vi "commander6.vi"() -> ()   [LabVIEW 2015]
uses:
  G_DATA.vi
  G_LCM.vi
  G_VEH.vi
  G_NAV.vi
  G_PATH.vi
  G_SEN.vi
  <vilib>/addons/control/pid/pid.llb/PID (DBL).vi
  <vilib>/addons/control/pid/NI_PID_pid.lvlib
panel:
  in  "handle":dbl
  in  "shifthold":dbl=0.0025
  out "String":string="콜 서비스 대기 중"
  out "EURECAR_VISION":T1
  out "count":i32
  out "P2V Sign":picture[](array[picture])=[bytes[7530], bytes[7530], bytes[7530], bytes[7530]]
  out "Array 2":picture[](array[picture])
  out "sign 2":picture[](array[picture])
  out "sign":picture[](array[picture])
  in  "TTL":bool
  in  "Steering gain":dbl=0.8
  out "obs shift":dbl format="%.2f"
  in  "lane keep":bool
  in  "replay":bool
  in  "x":dbl min=-5.0 max=5.0 step=1.0
  out "lane_shift":dbl=0.06529975046455076
  out "display":u32=10
  out "control":u32=10
  out "update":bool=TRUE
  in  "save lcm":bool
  out "LCM Recv Data":string="GGA_2\t266\rSDT_GPS_DATA\t268\rGGA_1\t268\rRMC_2\t259\rRMC_1\t262\rEYE_RAW_T\t537\rPATH_T\t1344\rIBEO_2202_T\t672\rPOS_T\t3572\rCON_T\t4009\rCAN_T\t4707\r"
  out "GPS DATA 2":T2={"type"="WAAS", "x_lcc"=-395.2637182511565, "y_lcc"=-852.8277788987846, "latdev"=0.99, "londev"=0.99, "sats"=11, "gps_l1_ranges"=0, "gps_l1_mask_ranges"=0, "gps_l2_mask_ranges"=0, "Heading"=151.74409645131422, "lon"=127.35651, "lat"=36.36776, "time"="15:03:34.8", "hgps"=151.54, "lag"=0.0, "MAP"="KAIST"} {"lag" format="%#_5g"; "hgps" format="%#_5g"; "lat" format="%#_11g"; "lon" format="%#_11g"; "Heading" format="%#_5g"; "latdev" format="%#_4g"; "londev" format="%#_4g"}
  in  "Obs":bool=TRUE
  in  "Log":bool
  out "path":u32=10
  out "sensor":u32=10 format="%02.0f"
  out "Speed limit":dbl=20.0
  out "collision":bool
  in  "Load Path":bool
  in  "Max. Vel.":dbl=20.0 min=-5.0 max=120.0 step=5.0
  in  "RESET PATH":bool
  out "col":i16(graph)
  out "stop":bool
  in  "Reverse":bool
  in  "STOP":bool
  out "Waveform Chart 4":cluster{"auto":i16, "run":i16}(graph)={"auto"=1, "run"=0}
  out "Waveform Chart 3":cluster{"Steer_input":dbl, dbl, "handle":dbl}(graph)
  out "Waveform Chart 2":T3(graph)={"VS_des"=0.0, "VS_can"=31.498562500000002, "VS_des"=20.0}
  out "Heading":cluster{"Heading":dbl, "hgps":dbl}(graph)={"Heading"=151.74409645131422, "hgps"=151.54}
  out "XY Graph 2":cluster{"Y":dbl[], "Y":dbl[]}[](graph)=[{"Y"=[-395.3040396828474], "Y"=[-852.7527551292769]}, {"Y"=array[29298 elements], "Y"=array[29298 elements]}, {"Y"=array[29298 elements], "Y"=array[29298 elements]}, {"Y"=[-390.58210518912017], "Y"=[-861.284610912867]}]
  out "Gauge":cluster{dbl, dbl, dbl}(knob)={0.0, 31.498562500000002, 20.0} scale=-20.0..140.0
  out "Meter":cluster{dbl, dbl, dbl}(knob)={-3.5333877271700453, -5.2, -7.217874503679048} scale=-550.0..550.0
  out "XY Graph":cluster{"Y":dbl[], "Y":dbl[]}[](graph)=[{"Y"=array[11233 elements], "Y"=array[11233 elements]}, {"Y"=[-0.0, 0.0027755521495791413, 0.011103235155417224, 0.024986130588096955, 0.04442938073793812, 0.0694401981527264, 0.10002787904836907, 0.13620382065079895, 0.17798154254490584, 0.22537671212434418, 0.2784071742547809, 0.3370929852830926, 0.40145645154536425, 0.4715221725490224, 0.5473170890276435, 0.6288705360921867, 0.7162143017295008, 0.8093826909282242, 0.9084125957438758, 1.0133435716494645, 1.1242179205557647, 1.2410807809266515, 1.3639802254602955, 1.4929673668571652, 1.6280964722509026, 1.769425086939485, 1.9170141681219874, 2.0709282294217246, 2.2312354970611636, 2.3980080786478197, 2.5713221456362234], "Y"=[0.0, 0.5, 1.0, 1.5, 2.0, 2.5, 3.0, 3.5, 4.0, 4.5, 5.0, 5.5, 6.0, 6.5, 7.0, 7.5, 8.0, 8.5, 9.0, 9.5, 10.0, 10.5, 11.0, 11.5, 12.0, 12.5, 13.0, 13.5, 14.0, 14.5, 15.0]}, {"Y"=[-0.40885366553013214], "Y"=[0.1442103688222703]}, {"Y"=array[212 elements], "Y"=array[212 elements]}, {"Y"=[-0.925, -0.925, -0.925, -0.6775, -0.6775, -0.925, -0.925, -0.925, -0.925, -0.6775, -0.6775, -0.925, -0.925, -0.925, 0.9025, 0.9025, 0.9025, 0.6775, 0.6775, 0.9025, 0.9025, 0.9025, 0.9025, 0.6775, 0.6775, 0.9025, 0.9025, 0.9025, -0.925], "Y"=[-0.75, -0.224, 0.224, 0.224, -0.224, -0.224, 0.224, 2.415, 2.885, 2.885, 2.415, 2.415, 2.885, 3.5, 3.5, 2.885, 2.415, 2.415, 2.885, 2.885, 2.415, 0.224, -0.224, -0.224, 0.224, 0.224, -0.224, -0.75, -0.75]}, {"Y"=[0.0, 0.0, 0.0, 0.0, 0.0, 0.0, 0.0, 0.0, 0.0, 0.0], "Y"=[0.0, 0.5, 1.0, 1.5, 2.0, 2.5, 3.0, 3.5, 4.0, 4.5]}, {"Y"=[1.41796875, 1.3798326583616436, 1.3415997434556484, 1.3032752327956258, 1.2648643538951874, 1.226372334267944, 1.1878044014275073, 1.1491657828874886, 1.110461706161499, 1.07169739876315], "Y"=[0.0, 0.5, 1.0, 1.5, 2.0, 2.5, 3.0, 3.5, 4.0, 4.5]}, {"Y"=[-2.5234375, -2.5105986626297234, -2.4915998479127883, -2.466420726940036, -2.4350409708023073, -2.3974402505904435, -2.3535982373952864, -2.303494602307677, -2.247109016418457, -2.184421150818467], "Y"=[0.0, 0.5, 1.0, 1.5, 2.0, 2.5, 3.0, 3.5, 4.0, 4.5]}, {"Y"=[0.0, 0.0, 0.0, 0.0, 0.0, 0.0, 0.0, 0.0, 0.0, 0.0, 0.0, 0.0, 0.0, 0.0, 0.0, 0.0, 0.0, 0.0, 0.0, 0.0], "Y"=[0.0, 0.5, 1.0, 1.5, 2.0, 2.5, 3.0, 3.5, 4.0, 4.5, 5.0, 5.5, 6.0, 6.5, 7.0, 7.5, 8.0, 8.5, 9.0, 9.5]}]
  in  "Make WPT":bool
  # "e"
  # "V2I Traffic Signal"
  # "CNN\nSign\nDetection"
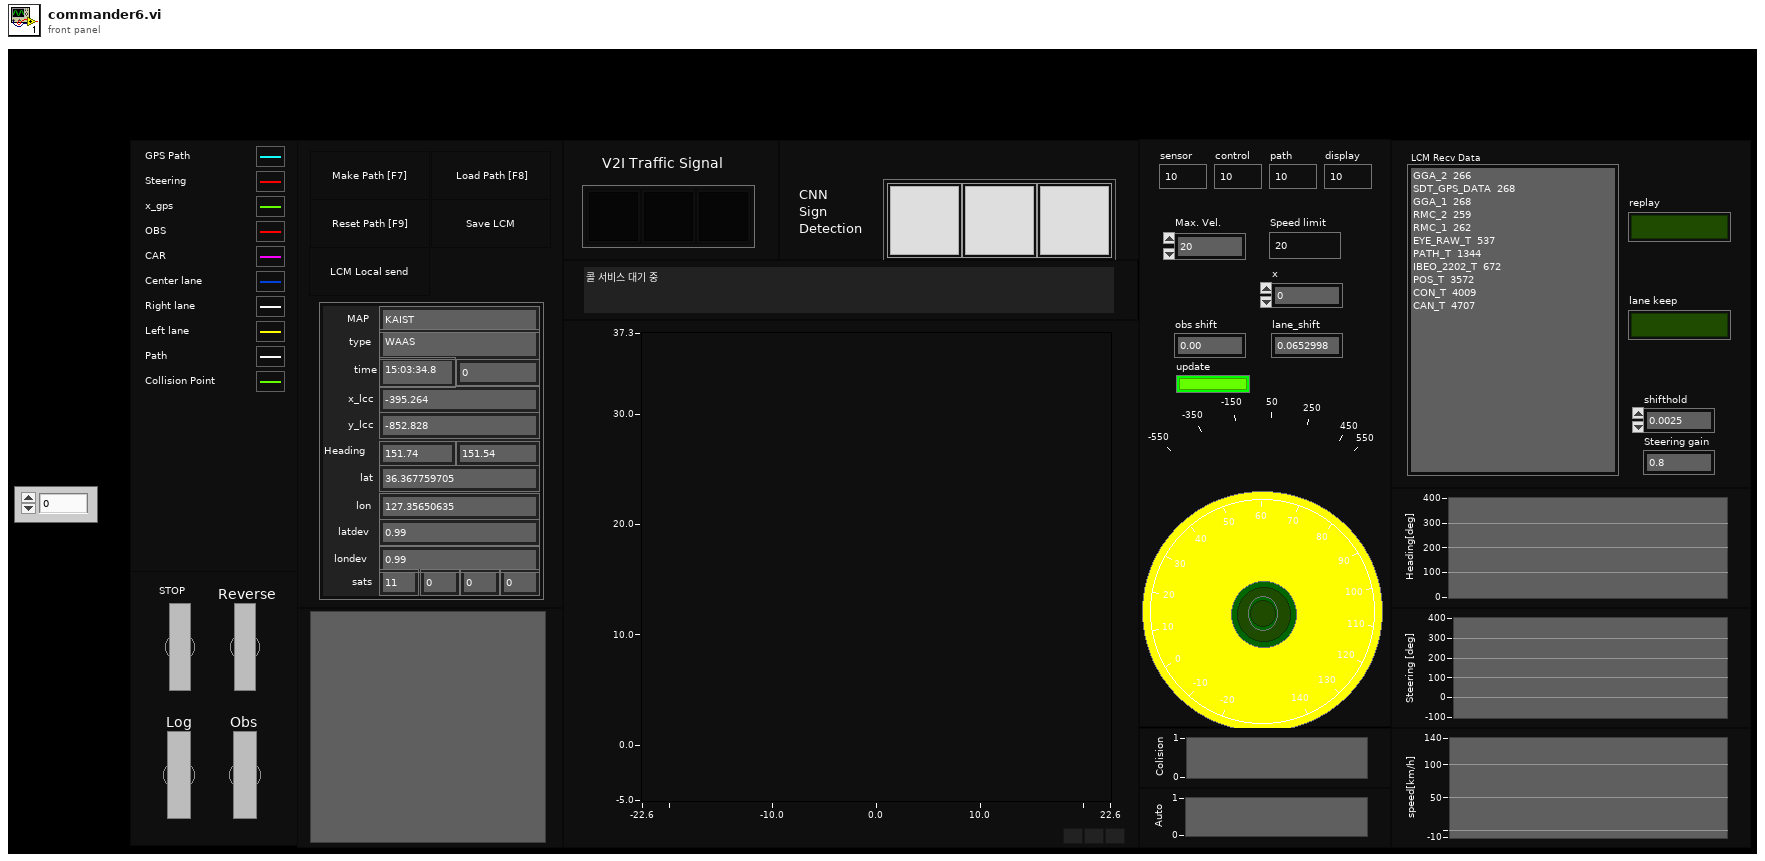
[diagram p1: front panel]
types:
  T1 = cluster{"hash":i64, "sys time":i64, "status":i32, "TS_num":i32, "TS_type":i32[], "TS_loc_x":dbl[], "TS_loc_y":dbl[]}
  T2 = cluster{"type":string, "x_lcc":dbl, "y_lcc":dbl, "latdev":sgl, "londev":sgl, "sats":u8, "gps_l1_ranges":u8, "gps_l1_mask_ranges":u8, "gps_l2_mask_ranges":u8, "Heading":dbl, "lon":sgl, "lat":sgl, "time":string, "hgps":dbl, "lag":dbl, "MAP":string}
  T3 = cluster{"VS_des":dbl, "VS_can":dbl, "VS_des":dbl}
  T4 = enum8{"Enabled", "Disabled", "Disabled and Grayed Out"}
  T5 = cluster{"proportional gain (Kc)":dbl, "integral time (Ti, min)":dbl, "derivative time (Td, min)":dbl}
  T6 = cluster{"idx":i32, "x":dbl, "y":dbl, "h":dbl, "x_path":dbl}
  T7 = cluster{"idx":i32, "x":dbl, "y":dbl, "hp":dbl, "x_path":dbl}
  T8 = cluster{"Steer_input":dbl, "Steer_output":dbl, "VS_des":dbl, "VS_can":dbl, "heading":dbl, "auto":bool, "run":bool, "x":dbl, "y":dbl}
  T9 = cluster{"X":cluster{"idx":i32, "x":dbl, "y":dbl, "h":dbl, "x_path":dbl}}[]
  T10 = typedef "imagedata.ctl" = cluster{"image type":i32, "image depth":i32, "image":u8[], "mask":u8[], "colors":u32[], "Rectangle":cluster{"left":i16, "top":i16, "right":i16, "bottom":i16}}
  T11 = cluster{"hash":i64, "sys time":i64, "s_lat":dbl, "s_lon":dbl, "d_lat":dbl, "d_lon":dbl, "Message":i64}
  T12 = cluster{"GPSTime":dbl, "attitude[2]":dbl, "lcc[0]":dbl, "lcc[1]":dbl, "heading_GPS":dbl}
  T13 = cluster{"Minimum":dbl, "Minimum":dbl, "Minimum":dbl, "Minimum":dbl, "Minimum":dbl}
  T14 = cluster{"X":cluster{"c_idx":i32, "xc":dbl, "yc":dbl, "hc":dbl, "xc_path":dbl}}[]
  T15 = cluster{"hash":i64, "sys time":i64, "time":dbl, "x":dbl, "y":dbl, "h":dbl, "numSV":i32, "postype":i32, "lag":i32, "hordev":dbl, "lat":dbl, "lon":dbl, "hgt":dbl, "map_idx":i32}
  T16 = cluster{"identifier":u32, "timestamp":timestamp, "payload":u8[]}
  T17 = cluster{"hash":i64, "sys time":i64, "size":i32, "data":u8[]}
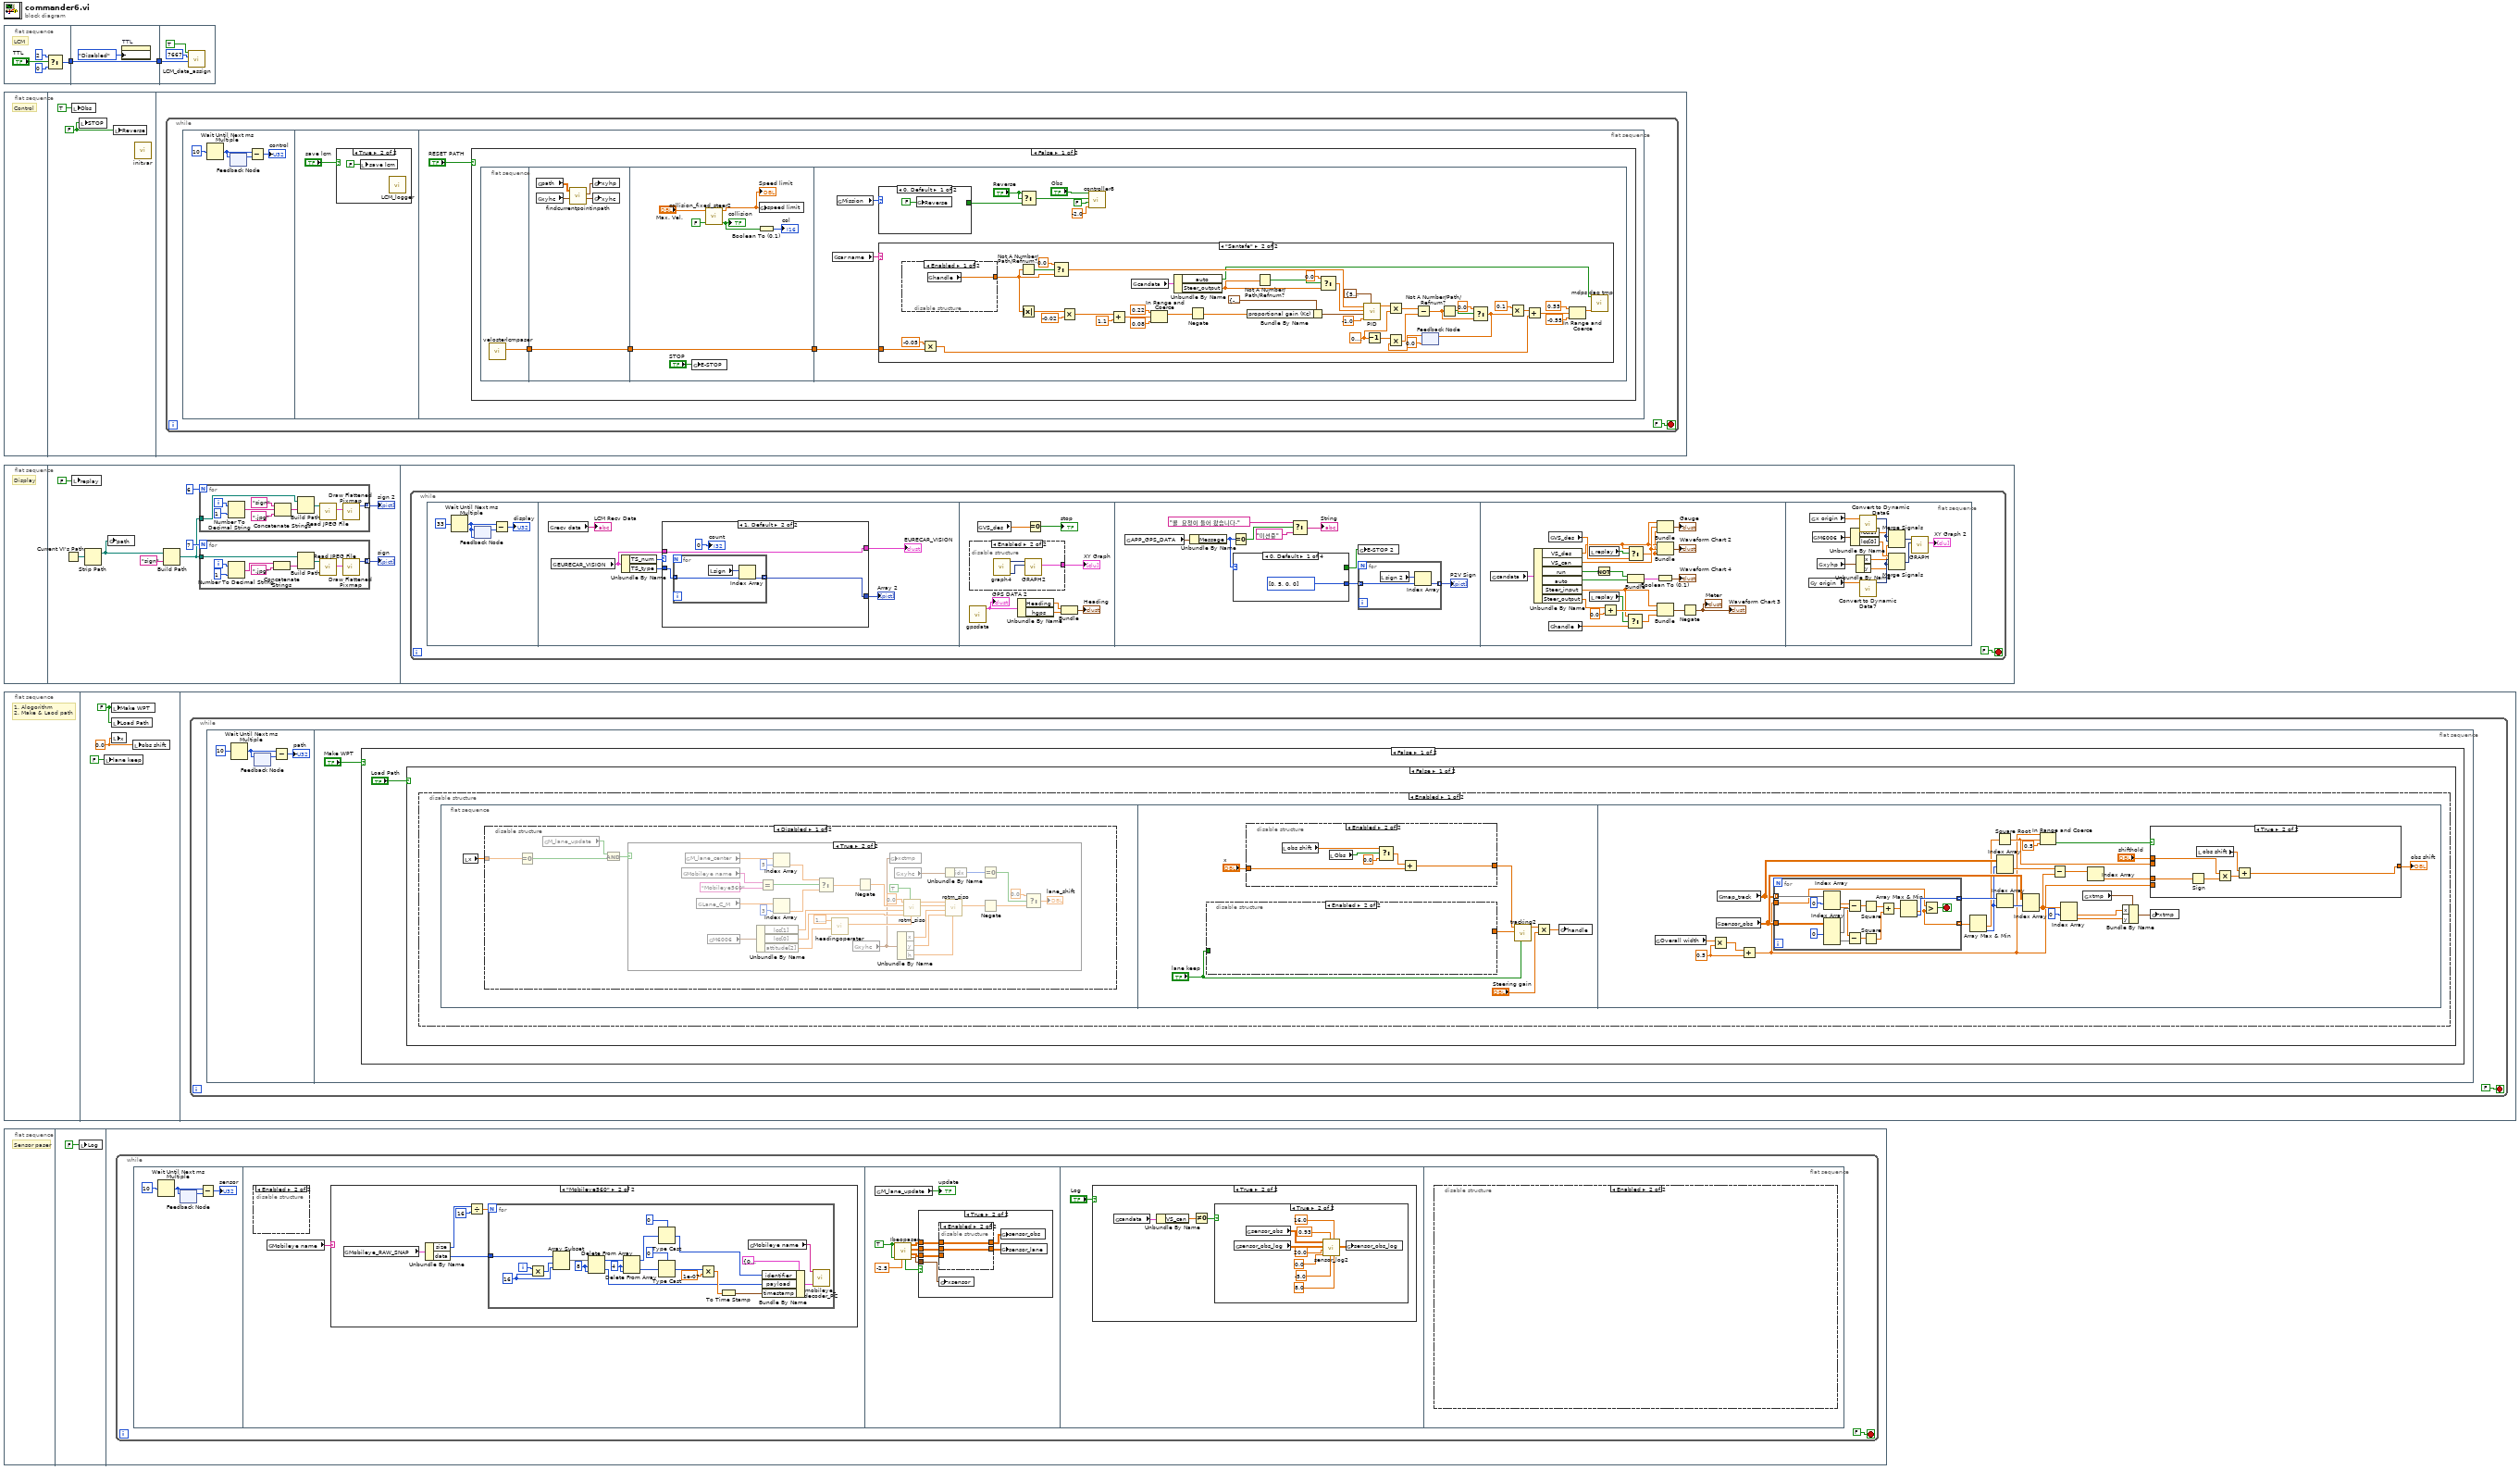
[diagram p0: block diagram]
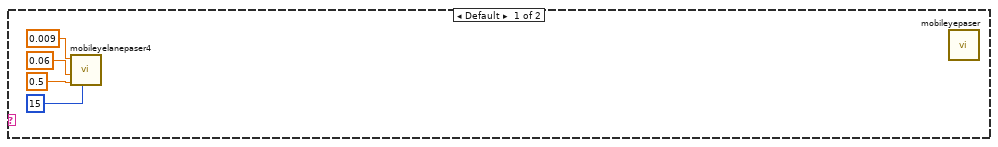
[diagram p2: hidden frame]
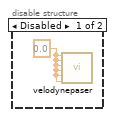
[diagram p3: hidden frame]
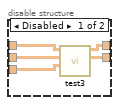
[diagram p5: hidden frame]
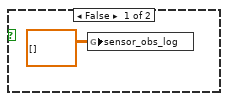
[diagram p6: hidden frame]
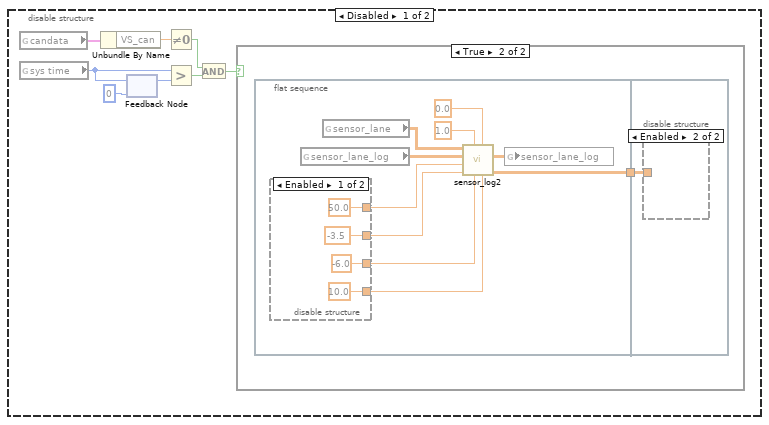
[diagram p8: hidden frame]
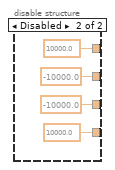
[diagram p10: hidden frame]
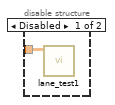
[diagram p11: hidden frame]
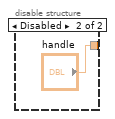
[diagram p14: hidden frame]
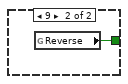
[diagram p15: hidden frame]
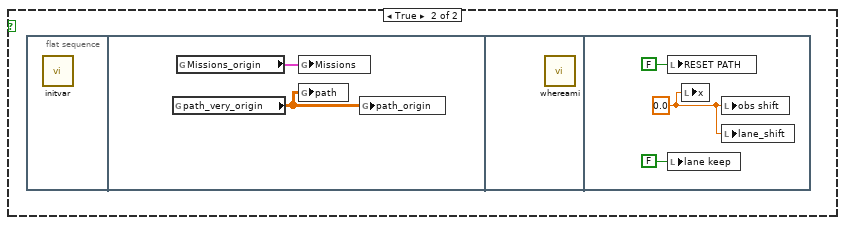
[diagram p16: hidden frame]
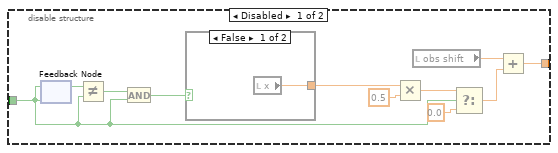
[diagram p19: hidden frame]
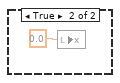
[diagram p20: hidden frame]
diagram:
  n1 = flat-sequence {
    tunnel: [w3] -> w1
    tunnel: [w8] -> w2
    tunnel: w1 -> [w8]
    tunnel: w2 -> [w11]
    frame #0 {
      # "LCM"
      n2 = Select(t=u16 2 ("time-to-live"), s="TTL", f=u16 0 ("time-to-live")) -> (s? t:f=w3:u16)
    }
    frame #1 {
      n3 = property on="TTL" class="Bool (strict)"("DisabledEnum"=T4."Disabled" ("Disabled")) -> ()  [unwired: 2 in, 2 out]
    }
    frame #2 {
      n4 = call "LCM_data_assign.vi"("time-to-live"=w11, "port"=u16 7667, "velodyne enable"=TRUE) -> ()  [unwired: 9 in]
    }
  }
  n5 = flat-sequence {
    frame #0 {
      # "Control"
    }
    frame #1 {
      w13 = FALSE ("LCM")
      n6 = local write "Obs"(TRUE ("obs")) -> ()
      n7 = local write "STOP"(w13) -> ()
      n8 = local write "Reverse"(w13) -> ()
      n9 = call "initvar.vi"() -> ()  [unwired: 12 in]
    }
    frame #2 {
      n10 = while {
        stop <- FALSE ("Loop 1") stop-if-true
        n11 = flat-sequence {
          frame #0 {
            n12 = Wait Until Next ms Multiple(millisecond multiple=u32 10 ("milliseconds to wait")) -> (millisecond timer value=w15:u32)
            n13 = feedback #1() -> (w16:u32)  [unwired: 1 in]
            n14 = feedback-in #1(w15) -> ()
            n15 = Subtract(x=w15, y=w16) -> (x-y=→"control":u32)
          }
          frame #1 {
            n16 = case shown="True" "save lcm" {
              frame False {
              }
              frame True {
                n17 = local write "save lcm"(FALSE ("save lcm")) -> ()
                n18 = call "LCM_logger.vi"() -> ()  [unwired: 12 in]
              }
            }
          }
          frame #2 {
            n19 = case shown="False" "RESET PATH" {
              frame False {
                n20 = flat-sequence {
                  tunnel: [w25] -> w24
                  tunnel: w24 -> [w26]
                  tunnel: [w26] -> w23
                  tunnel: w23 -> [w32]
                  tunnel: [w32] -> w22
                  tunnel: w22 -> [w40]
                  frame #0 {
                    n21 = call "velosterlcmpaser.vi"() -> ("mdps torque"=w25:dbl)  [unwired: 10 in, 1 out]
                  }
                  frame #1 {
                    n22 = global read "G_PATH.vi" "path"() -> (w28:dbl[][])
                    n23 = global read "G_VEH.vi" "xyhc"() -> (w29:T6)
                    n24 = call "findcurrentpointinpath.vi"("xyhc_in"=w29, "path_updated"=w28) -> ("xyhc_out"=w27:T6, "xyhp"=w30:T7)  [unwired: 8 in]
                    n25 = global write "G_VEH.vi" "xyhp"(w30) -> ()
                    n26 = global write "G_VEH.vi" "xyhc"(w27) -> ()
                  }
                  frame #2 {
                    n27 = global write "G_VEH.vi" "E-STOP"("STOP") -> ()
                    n28 = call "collision_fixed_steer2.vi"("obsclose"=FALSE, "Max. Vel."="Max. Vel.") -> ("collision"=w33:bool, "speed limit"=w31:dbl)  [unwired: 8 in]
                    "collision" <- w33
                    "Speed limit" <- w31
                    n29 = Boolean To (0,1)(Boolean=w33) -> (0, 1=→"col":i16)
                    n30 = global write "G_VEH.vi" "speed limit"(w31) -> ()
                  }
                  frame #3 {
                    n31 = global read "G_LCM.vi" "car name"() -> (w41:string)
                    n32 = global read "G_PATH.vi" "Mission"() -> (w46:i32)
                    n33 = case shown="0, Default" w46 {
                      tunnel: [_ w93] -> w43
                      frame 0, Default {
                        n34 = global write "G_VEH.vi" "Reverse"(FALSE ("Reverse")) -> ()
                      }
                      frame 9 {
                        n35 = global read "G_VEH.vi" "Reverse"() -> (w93:bool)
                      }
                    }
                    n36 = case shown="\"Santafe\"" w41 {
                      tunnel: w40 -> [_ w80]
                      frame "False", Default {
                      }
                      frame "Santafe" {
                        w69 = 0.6000000000000001 ("y")
                        n37 = disable-structure shown="Enabled" {
                          disable-tunnel: [w90 "handle"] -> w47
                          frame Enabled {
                            n38 = global read "G_VEH.vi" "handle"() -> (w90:dbl)
                          }
                          frame Disabled {
                          }
                        }
                        n39 = Multiply(x=-0.05 ("x 5"), y=w80) -> (x*y=w78:dbl)
                        n40 = Not A Number/Path/Refnum?(number/path/refnum=w47) -> (NaN/Path/Refnum?=w72:bool)
                        n41 = Absolute Value(x=w47) -> (abs(x)=w63:dbl)
                        n42 = Select(t=0.0, s=w72, f=w47) -> (s? t:f=w71:dbl)
                        n43 = Multiply(x=w63, y=-0.02) -> (x*y=w61:dbl)
                        n44 = Add(x=w61, y=1.1) -> (x+y=w59:dbl)
                        n45 = global read "G_VEH.vi" "candata"() -> (w89:T8)
                        n46 = In Range and Coerce(upper limit=0.22, x=w59, lower limit=0.08) -> (coerced(x)=w56:dbl)  [unwired: 1 out]
                        n47 = Unbundle By Name(w89) -> ("auto"=w48:bool, "Steer_output"=w75:dbl)
                        n48 = Negate(x=w56) -> (-x=w54:dbl)
                        n49 = Bundle By Name(cluster=T5 {"proportional gain (Kc)"=-0.1, "integral time (Ti, min)"=0.0, "derivative time (Td, min)"=0.0} ("PID gains"), "proportional gain (Kc)"=w54) -> (w53:T5)
                        n50 = Not A Number/Path/Refnum?(number/path/refnum=w75) -> (NaN/Path/Refnum?=w77:bool)
                        n51 = Select(t=0.0, s=w77, f=w75) -> (s? t:f=w74:dbl)
                        n52 = call-poly <vilib>:"PID.vi"("output range"=cluster{"output high":dbl, "output low":dbl} {"output high"=5.0, "output low"=-5.0}, "dt (s)"=-1.0, "PID gains"=w53, "process variable"=w74, "setpoint"=w71) -> ("output"=w70:dbl)  [unwired: 5 in, 1 out]
                        n53 = Decrement(x=w69) -> (x-1=w68:dbl)
                        n54 = Multiply(x=w70, y=w69) -> (x*y=w65:dbl)
                        n55 = feedback #2(0.0) -> (w67:dbl)
                        n56 = Multiply(x=w68, y=w67) -> (x*y=w66:dbl)
                        n57 = Subtract(x=w65, y=w66) -> (x-y=w50:dbl)
                        n58 = Not A Number/Path/Refnum?(number/path/refnum=w50) -> (NaN/Path/Refnum?=w52:bool)
                        n59 = Select(t=0.0, s=w52, f=w50) -> (s? t:f=w49:dbl)
                        n60 = feedback-in #2(w49) -> ()
                        n61 = Multiply(x=0.1 ("x 2"), y=w49) -> (x*y=w79:dbl)
                        n62 = Add(x=w79, y=w78) -> (x+y=w86:dbl)
                        n63 = In Range and Coerce(upper limit=0.55, x=w86, lower limit=-0.55) -> (coerced(x)=w85:dbl)  [unwired: 1 out]
                        n64 = call "mdps daq tmp.vi"("steering"=w85, "auto"=w48) -> ()  [unwired: 10 in]
                      }
                    }
                    n65 = Select(t="Reverse", s="Reverse", f=w43) -> (s? t:f=w44:bool)
                    n66 = call "controller8.vi"("Neg max speed"=-2.0, "vel"=FALSE, "reverse"=w44, "obs"="Obs") -> ()  [unwired: 8 in]
                  }
                }
              }
              frame True {
                n67 = flat-sequence {
                  frame #0 {
                    n68 = call "initvar.vi"() -> ()  [unwired: 12 in]
                  }
                  frame #1 {
                    n69 = global read "G_PATH.vi" "path_very_origin"() -> (w95:dbl[][])
                    n70 = global read "G_PATH.vi" "Missions_origin"() -> (w94:T9)
                    n71 = global write "G_PATH.vi" "Missions"(w94) -> ()
                    n72 = global write "G_PATH.vi" "path"(w95) -> ()
                    n73 = global write "G_PATH.vi" "path_origin"(w95) -> ()
                  }
                  frame #2 {
                    n74 = call "whereami.vi"() -> ()  [unwired: 12 in]
                  }
                  frame #3 {
                    w96 = 0.0 ("x")
                    n75 = local write "RESET PATH"(FALSE ("RESET PATH")) -> ()
                    n76 = local write "lane keep"(FALSE ("lane keep")) -> ()
                    n77 = local write "x"(w96) -> ()
                    n78 = local write "obs shift"(w96) -> ()
                    n79 = local write "lane_shift"(w96) -> ()
                  }
                }
              }
            }
          }
        }
      }
    }
  }
  n80 = flat-sequence {
    frame #0 {
      # "Display"
    }
    frame #1 {
      n81 = Current VI's Path() -> (path=w106:path)
      n82 = local write "replay"(FALSE ("replay")) -> ()
      n83 = Strip Path(path=w106) -> (stripped path=w99:path)  [unwired: 1 out]
      n84 = global write "G_DATA.vi" "path"(w99) -> ()
      n85 = Build Path(base path=w99, name or relative path="sign") -> (appended path=w100:path)
      n86 = for {
        N: 6 -> [_]
        tunnel: [w116] -> w102 mode=indexing
        tunnel: w100 -> [w111]
        i -> [w115]
        n87 = Number To Decimal String(number=w115, width (-)=i16 1) -> (decimal integer string=w113:string)
        n88 = Concatenate Strings("sign" ("string"), w113, ".jpg") -> (w110:string)
        n89 = Build Path(base path=w111, name or relative path=w110) -> (appended path=w109:path)
        n90 = call <vilib>:"Read JPEG File.vi"("path to JPEG file"=w109) -> ("image data"=w117:T10)  [unwired: 8 in, 2 out]
        n91 = call <vilib>:"Draw Flattened Pixmap.vi"("image data"=w117) -> ("new picture"=w116:picture)  [unwired: 8 in]
      }
      "sign 2" <- w102
      n92 = for {
        N: 7 -> [_]
        tunnel: [w125] -> w103 mode=indexing
        tunnel: w100 -> [w120]
        i -> [w124]
        n93 = Number To Decimal String(number=w124, width (-)=i16 1) -> (decimal integer string=w122:string)
        n94 = Concatenate Strings(w122, ".jpg") -> (w119:string)
        n95 = Build Path(base path=w120, name or relative path=w119) -> (appended path=w118:path)
        n96 = call <vilib>:"Read JPEG File.vi"("path to JPEG file"=w118) -> ("image data"=w126:T10)  [unwired: 8 in, 2 out]
        n97 = call <vilib>:"Draw Flattened Pixmap.vi"("image data"=w126) -> ("new picture"=w125:picture)  [unwired: 8 in]
      }
      "sign" <- w103
    }
    frame #2 {
      n98 = while {
        stop <- FALSE ("Loop 2") stop-if-true
        n99 = flat-sequence {
          frame #0 {
            n100 = Wait Until Next ms Multiple(millisecond multiple=u32 33 ("milliseconds to wait")) -> (millisecond timer value=w128:u32)
            n101 = feedback #3(w128) -> (w130:u32)
            n102 = feedback-in #3(w128) -> ()
            n103 = Subtract(x=w128, y=w130) -> (x-y=→"display":u32)
          }
          frame #1 {
            n104 = global read "G_LCM.vi" "recv data"() -> (→"LCM Recv Data":string)
            n105 = global read "G_LCM.vi" "EURECAR_VISION"() -> (w134:T1)
            n106 = Unbundle By Name(w134) -> ("TS_num"=w137:i32, "TS_type"=w136:i32[])
            n107 = case shown="1, Default" w137 {
              tunnel: w136 -> [_ w152]
              tunnel: [w145 w151] -> w135
              tunnel: w134 -> [_ w149]
              tunnel: [w138 w149] -> w133
              frame 0 {
                w147 = 100 ("x")
                n108 = local read "count"() -> (w148:i32)
                n109 = Increment(x=w148) -> (x+1=w143:i32)
                n110 = Max & Min(x=w147, y=w143) -> (min(x,y)=w142:i32)  [unwired: 1 out]
                n111 = local read "EURECAR_VISION"() -> (w139:T1)
                n112 = local write "count"(w142) -> ()
                n113 = Equal?(x=w147, y=w142) -> (x = y?=w141:bool)
                n114 = local read "Array 2"() -> (w144:picture[])
                n115 = Select(t=T1 {"hash"=0, "sys time"=0, "status"=0, "TS_num"=0, "TS_type"=[], "TS_loc_x"=[], "TS_loc_y"=[]} ("EURECAR_VISION"), s=w141, f=w139) -> (s? t:f=w138:T1)
                n116 = Select(t=picture[] [], s=w141, f=w144) -> (s? t:f=w145:picture[])
              }
              frame 1, Default {
                n117 = for {
                  tunnel: w152 -> [w154] mode=indexing
                  tunnel: [w153] -> w151 mode=indexing
                  n118 = local read "sign"() -> (w155:picture[])
                  n119 = Index Array(array=w155, index=w154) -> (element=w153:picture)
                }
                "count" <- 0 ("Numeric Control")
              }
            }
            "Array 2" <- w135
            "EURECAR_VISION" <- w133
          }
          frame #2 {
            n120 = disable-structure shown="Enabled" {
              disable-tunnel: [w163 w167] -> w156
              frame Disabled {
                n121 = call "graph3.vi"("replay"="replay") -> ("XY Graph"=w163:cluster{"Y":dbl[], "Y":dbl[]}[])  [unwired: 9 in, 1 out]
              }
              frame Enabled {
                n122 = call "graph4.vi"() -> ("y"=w165:dynamicdata, "x"=w166:dynamicdata)  [unwired: 10 in]
                n123 = call "GRAPH2"("Y Input"=w165, "X Input"=w166) -> ("XY Graph"=w167:cluster{"Y":dbl[], "Y":dbl[]}[])  [unwired: 3 in, 6 out]
              }
            }
            "XY Graph" <- w156
            n124 = call "gpsdata.vi"() -> ("GPS DATA 2"=w158:T2)  [unwired: 11 in]
            "GPS DATA 2" <- w158
            n125 = global read "G_VEH.vi" "VS_des"() -> (w162:dbl)
            n126 = Unbundle By Name(w158) -> ("Heading"=w160:dbl, "hgps"=w159:dbl)
            n127 = Equal To 0?(x=w162) -> (x = 0?=→"stop":bool)
            n128 = Bundle("Heading"=w160, "hgps"=w159) -> (→"Heading":cluster{"Heading":dbl, "hgps":dbl})  [unwired: 1 in]
          }
          frame #3 {
            n129 = global read "G_LCM.vi" "APP_GPS_DATA"() -> (w173:T11)
            n130 = Unbundle By Name(w173) -> ("Message"=w172:i64)
            n131 = Equal To 0?(x=w172) -> (x = 0?=w171:bool)
            n132 = case shown="0, Default" w172 {
              tunnel: [_ TRUE _ _] -> w176
              tunnel: [i32[] [0, 5, 0, 0] i32[] [1, 5, 0, 0] i32[] [0, 2, 0, 0] i32[] [0, 5, 3, 0]] -> w175
              frame 0, Default {
              }
              frame 1 {
              }
              frame 2 {
              }
              frame 3 {
              }
            }
            n133 = Select(t="콜  요청이 들어 왔습니다.", s=w171, f="미션중") -> (s? t:f=→"String":string)
            n134 = global write "G_VEH.vi" "E-STOP 2"(w176) -> ()
            n135 = for {
              tunnel: w175 -> [w183] mode=indexing
              tunnel: [w182] -> w174 mode=indexing
              n136 = local read "sign 2"() -> (w184:picture[])
              n137 = Index Array(array=w184, index=w183) -> (element=w182:picture)
            }
            "P2V Sign" <- w174
          }
          frame #4 {
            n138 = global read "G_VEH.vi" "candata"() -> (w206:T8)
            n139 = Unbundle By Name(w206) -> ("VS_des"=w187:dbl, "VS_can"=w199:dbl, "run"=w197:bool, "auto"=w198:bool, "Steer_input"=w191:dbl, "Steer_output"=w196:dbl)
            n140 = global read "G_VEH.vi" "VS_des"() -> (w188:dbl)
            n141 = global read "G_VEH.vi" "handle"() -> (w192:dbl)
            n142 = local read "replay"() -> (w189:bool)
            n143 = local read "replay"() -> (w193:bool)
            n144 = Not(x=w197) -> (.not. x?=w201:bool)
            n145 = Add(x=w196, y=0.0) -> (x+y=w194:dbl)
            n146 = Select(t=w191, s=w193, f=w192) -> (s? t:f=w190:dbl)
            n147 = Select(t=w187, s=w189, f=w188) -> (s? t:f=w186:dbl)
            n148 = Bundle(w201, "auto"=w198) -> (w203:cluster{bool, "auto":bool})  [unwired: 1 in]
            n149 = Boolean To (0,1)(Boolean=w203) -> (0, 1=→"Waveform Chart 4":cluster{i16, "auto":i16})
            n150 = Bundle("VS_des"=w187, "VS_can"=w199, "VS_des"=w186) -> (→"Gauge":T3)  [unwired: 1 in]
            n151 = Bundle("VS_des"=w187, "VS_can"=w199, "VS_des"=w186) -> (→"Waveform Chart 2":T3)  [unwired: 1 in]
            n152 = Bundle("Steer_input"=w191, w194, "handle"=w190) -> (w205:cluster{"Steer_input":dbl, dbl, "handle":dbl})  [unwired: 1 in]
            n153 = Negate(x=w205) -> (-x=→"Meter" →"Waveform Chart 3":cluster{"Steer_input":dbl, dbl, "handle":dbl})
          }
          frame #5 {
            n154 = global read "G_PATH.vi" "y origin"() -> (w210:dbl[])
            n155 = global read "G_PATH.vi" "x origin"() -> (w211:dbl[])
            n156 = global read "G_NAV.vi" "M6006"() -> (w215:T12)
            n157 = global read "G_VEH.vi" "xyhp"() -> (w209:T6)
            n158 = Unbundle By Name(w215) -> ("lcc[1]"=w216:dbl, "lcc[0]"=w217:dbl)
            n159 = Unbundle By Name(w209) -> ("x"=w213:dbl, "y"=w212:dbl)
            n160 = call "Convert to Dynamic Data6"("Array"=w211) -> ("Dynamic Data Type"=w219:dynamicdata)  [unwired: 3 in]
            n161 = call "Convert to Dynamic Data7"("Array"=w210) -> ("Dynamic Data Type"=w218:dynamicdata)  [unwired: 3 in]
            n162 = Merge Signals(w216, w219, w219, w213) -> (w208:dynamicdata)
            n163 = Merge Signals(w217, w218, w218, w212) -> (w207:dynamicdata)
            n164 = call "GRAPH"("Y Input"=w207, "X Input"=w208) -> ("XY Graph"=→"XY Graph 2":cluster{"Y":dbl[], "Y":dbl[]}[])  [unwired: 3 in, 6 out]
          }
        }
      }
    }
  }
  n165 = flat-sequence {
    frame #0 {
      # "1. Alogorithm\n2. Make & Laod path"
    }
    frame #1 {
      w220 = 0.0 ("x")
      w222 = FALSE ("Make WPT")
      n166 = local write "lane keep"(FALSE ("lane update")) -> ()
      n167 = local write "Make WPT"(w222) -> ()
      n168 = local write "Load Path"(w222) -> ()
      n169 = local write "x"(w220) -> ()
      n170 = local write "obs shift"(w220) -> ()
    }
    frame #2 {
      n171 = while {
        stop <- FALSE ("Loop 3") stop-if-true
        n172 = flat-sequence {
          frame #0 {
            n173 = Wait Until Next ms Multiple(millisecond multiple=u32 10 ("milliseconds to wait")) -> (millisecond timer value=w224:u32)
            n174 = feedback #4() -> (w226:u32)  [unwired: 1 in]
            n175 = feedback-in #4(w224) -> ()
            n176 = Subtract(x=w224, y=w226) -> (x-y=→"path":u32)
          }
          frame #1 {
            n177 = case shown="False" "Make WPT" {
              frame False {
                n178 = case shown="False" "Load Path" {
                  frame False {
                    n179 = disable-structure shown="Enabled" {
                      frame Enabled {
                        n180 = flat-sequence {
                          frame #0 {
                            n181 = local read "x"() -> (w230:dbl)
                            n182 = disable-structure shown="Disabled" {
                              disable-tunnel: w230 -> [w231 _]
                              frame Disabled {
                                n183 = Equal To 0?(x=w231) -> (x = 0?=w232:bool)
                                n184 = global read "G_SEN.vi" "M_lane_update"() -> (w233:bool)
                                n185 = And(x=w233, y=w232) -> (x .and. y?=w234:bool)
                                n186 = case shown="True" w234 {
                                frame False {
                                }
                                frame True {
                                n187 = global read "G_LCM.vi" "Mobileye name"() -> (w242:string)
                                n188 = global read "G_SEN.vi" "M_lane_center"() -> (w237:dbl[])
                                n189 = global read "G_SEN.vi" "Lane_C_M"() -> (w266:dbl[])
                                n190 = global read "G_NAV.vi" "M6006"() -> (w263:T12)
                                n191 = Unbundle By Name(w263) -> ("lcc[1]"=w262:dbl, "lcc[0]"=w261:dbl, "attitude[2]"=w259:dbl)
                                n192 = Equal?(x=w242, y="Mobileye560") -> (x = y?=w240:bool)
                                n193 = Index Array(array=w237, index=5) -> (element=w236:dbl)
                                n194 = Index Array(array=w266, index=3) -> (element=w239:dbl)
                                n195 = Select(t=w236, s=w240, f=w239) -> (s? t:f=w235:dbl)
                                n196 = call "headingoperater.vi"("h1"=w259, "h2"=1.5707963267948966) -> ("h2-h1"=w258:dbl)  [unwired: 8 in, 1 out]
                                n197 = global read "G_VEH.vi" "xyhc"() -> (w243:T6)
                                n198 = Negate(x=w235) -> (-x=w257:dbl)
                                n199 = global write "G_VEH.vi" "xctmp"(w243) -> ()
                                n200 = global read "G_VEH.vi" "xyhc"() -> (w264:T6)
                                n201 = Unbundle By Name(w243) -> ("x"=w252:dbl, "y"=w251:dbl, "h"=w250:dbl)
                                n202 = call "rotm_siso.vi"("angle[rad]"=w258, "reverse"=TRUE, "y0"=w261, "x0"=w262, "y"=w257, "x"=0.0) -> ("y'"=w253:dbl, "x'"=w254:dbl)  [unwired: 4 in]
                                n203 = Unbundle By Name(w264) -> ("idx"=w248:i32)
                                n204 = call "rotm_siso.vi"("angle[rad]"=w250, "y0"=w251, "x0"=w252, "y"=w253, "x"=w254) -> ("y'"=w249:dbl)  [unwired: 5 in, 1 out]
                                n205 = Equal To 0?(x=w248) -> (x = 0?=w247:bool)
                                n206 = Negate(x=w249) -> (-x=w244:dbl)
                                n207 = Select(t=0.0, s=w247, f=w244) -> (s? t:f=→"lane_shift":dbl)
                                }
                                }
                              }
                              frame Enabled {
                              }
                            }
                          }
                          frame #1 {
                            n208 = disable-structure shown="Enabled" {
                              disable-tunnel: [w279 _] -> w272
                              disable-tunnel: "lane keep" -> [w275 _]
                              frame Disabled {
                                n209 = feedback #5(w275) -> (w276:bool)
                                n210 = feedback-in #5(w275) -> ()
                                n211 = Not Equal?(x=w276, y=w275) -> (x != y?=w274:bool)
                                n212 = And(x=w274, y=w275) -> (x .and. y?=w278:bool)
                                n213 = case shown="False" w278 {
                                tunnel: [w285 _] -> w277
                                frame False {
                                n214 = local read "x"() -> (w285:dbl)
                                }
                                frame True {
                                n215 = local write "x"(0.0 ("x")) -> ()
                                }
                                }
                                n216 = Multiply(x=w277, y=0.5) -> (x*y=w283:dbl)
                                n217 = local read "obs shift"() -> (w280:dbl)
                                n218 = Select(t=w283, s=w275, f=0.0) -> (s? t:f=w281:dbl)
                                n219 = Add(x=w280, y=w281) -> (x+y=w279:dbl)
                              }
                              frame Enabled {
                              }
                            }
                            n220 = disable-structure shown="Enabled" {
                              disable-tunnel: [w297 w298] -> w273
                              disable-tunnel: "x" -> [w290 w299]
                              frame Disabled {
                                w292 = 0.98 ("Shift LPF gain")
                                n221 = Multiply(x=w290, y=0.5) -> (x*y=w289:dbl)
                                n222 = local read "lane_shift"() -> (w288:dbl)
                                n223 = Add(x=w288, y=w289) -> (x+y=w287:dbl)
                                n224 = feedback #6(w287) -> (w293:dbl)
                                n225 = Decrement(x=w292) -> (x-1=w294:dbl)
                                n226 = Multiply(x=w293, y=w292) -> (x*y=w295:dbl)
                                n227 = Multiply(x=w294, y=w287) -> (x*y=w296:dbl)
                                n228 = Subtract(x=w295, y=w296) -> (x-y=w297:dbl)
                                n229 = feedback-in #6(w297) -> ()
                              }
                              frame Enabled {
                                n230 = local read "obs shift"() -> (w302:dbl)
                                n231 = local read "Obs"() -> (w303:bool)
                                n232 = Select(t=w302, s=w303, f=0.0) -> (s? t:f=w300:dbl)
                                n233 = Add(x=w300, y=w299) -> (x+y=w298:dbl)
                              }
                            }
                            n234 = call "tracking2.vi"("lane keep"="lane keep", "xbody"=w272, "xt"=w273) -> ("handle"=w269:dbl)  [unwired: 7 in, 1 out]
                            n235 = Multiply(x=w269, y="Steering gain") -> (x*y=w271:dbl)
                            n236 = global write "G_VEH.vi" "handle"(w271) -> ()
                          }
                          frame #2 {
                            w305 = 0.5 ("y")
                            n237 = global read "G_VEH.vi" "Overall width"() -> (w307:dbl)
                            n238 = Multiply(x=w307, y=w305) -> (x*y=w306:dbl)
                            n239 = global read "G_SEN.vi" "sensor_obs"() -> (w321:dbl[][])
                            n240 = global read "G_PATH.vi" "map_track"() -> (w320:dbl[][])
                            n241 = Add(x=w306, y=w305) -> (x+y=w304:dbl)
                            n242 = for {
                              tunnel: w320 -> [w367] mode=indexing
                              tunnel: w321 -> [w369]
                              tunnel: [w355] -> w327 mode=indexing
                              tunnel: [w356] -> w328 mode=indexing
                              tunnel: w304 -> [w353]
                              stop <- w354 stop-if-true
                              n243 = Index Array(array=w367, index #1=0 ("index")) -> (element #1=w365:dbl, element #2=w363:dbl)  [unwired: 1 in]
                              n244 = Index Array(array=w369, index (col) #1=0 ("disabled index (col)")) -> (element #1=w364:dbl[], element #2=w362:dbl[])  [unwired: 3 in]
                              n245 = Subtract(x=w365, y=w364) -> (x-y=w361:dbl[])
                              n246 = Subtract(x=w363, y=w362) -> (x-y=w360:dbl[])
                              n247 = Square(x=w361) -> (x^2=w359:dbl[])
                              n248 = Square(x=w360) -> (x^2=w358:dbl[])
                              n249 = Add(x=w359, y=w358) -> (x+y=w357:dbl[])
                              n250 = Array Max & Min(array=w357) -> (min value=w355:dbl, min index (indices)=w356:i32)  [unwired: 2 out]
                              n251 = Greater?(x=w353, y=w355) -> (0:w354:bool)
                            }
                            n252 = Array Max & Min(array=w327) -> (min value=w314:dbl, min index (indices)=w319:i32)  [unwired: 2 out]
                            n253 = Square Root(x=w314) -> (sqrt(x)=w310:dbl)
                            n254 = Index Array(array=w320, index (row)=w319) -> (element=w318:dbl[])  [unwired: 1 in]
                            n255 = Index Array(array=w328, index=w319) -> (element=w324:i32)
                            n256 = Index Array(array=w321, index (row)=w324) -> (element=w316:dbl[])  [unwired: 1 in]
                            n257 = In Range and Coerce(upper limit=w304, x=w310, lower limit=0.5) -> (In Range?=w312:bool)  [unwired: 1 out]
                            n258 = Subtract(x=w318, y=w316) -> (x-y=w315:dbl[])
                            n259 = Index Array(array=w316, index #1=0 ("index")) -> (element #1=w317:dbl, element #2=w322:dbl)  [unwired: 1 in]
                            n260 = global read "G_VEH.vi" "xtmp"() -> (w325:T6)
                            n261 = Index Array(array=w315) -> (element=w311:dbl)  [unwired: 1 in]
                            n262 = Bundle By Name(cluster=w325, "x"=w317, "y"=w322) -> (w326:T6)
                            n263 = case shown="True" w312 {
                              tunnel: w311 -> [_ w352]
                              tunnel: [w344 w349] -> w309
                              tunnel: w310 -> [w346 _]
                              tunnel: "shifthold" -> [w330 w348]
                              tunnel: w304 -> [w329 _]
                              frame False {
                                n264 = local read "obs shift"() -> (w341:dbl)
                                n265 = Multiply(x=w329, y=0.1) -> (x*y=w333:dbl)
                                n266 = Add(x=w329, y=w333) -> (x+y=w332:dbl)
                                n267 = Negate(x=w330) -> (-x=w331:dbl)
                                n268 = Sign(1:w341) -> (0:w343:dbl)
                                n269 = Greater?(x=w346, y=w332) -> (0:w345:bool)
                                n270 = Multiply(x=w343, y=w331) -> (x*y=w342:dbl)
                                n271 = Add(x=w341, y=w342) -> (x+y=w337:dbl)
                                n272 = Absolute Value(x=w337) -> (abs(x)=w340:dbl)
                                n273 = Greater?(x=w340, y=0.01) -> (0:w338:bool)
                                n274 = Select(t=w337, s=w338, f=0.0) -> (s? t:f=w335:dbl)
                                n275 = Select(t=w335, s=w345, f=w341) -> (s? t:f=w344:dbl)
                              }
                              frame True {
                                n276 = Sign(1:w352) -> (0:w347:dbl)
                                n277 = local read "obs shift"() -> (w350:dbl)
                                n278 = Multiply(x=w348, y=w347) -> (x*y=w351:dbl)
                                n279 = Add(x=w350, y=w351) -> (x+y=w349:dbl)
                              }
                            }
                            "obs shift" <- w309
                            n280 = global write "G_VEH.vi" "xtmp"(w326) -> ()
                          }
                        }
                      }
                      frame Disabled {
                      }
                    }
                  }
                  frame True {
                    n281 = flat-sequence {
                      frame #0 {
                        w371 = FALSE ("X Scale.Loose Fit")
                        w370 = u8 0 ("X Scale.Scale Fit")
                        n282 = call "initvar.vi"() -> ()  [unwired: 12 in]
                        n283 = property on="XY Graph" class="XYGraph (strict)"("XScale.ScaleFit"=w370, "YScale.ScaleFit"=w370, "XScale.LooseFit"=w371, "YScale.LooseFit"=w371) -> ()  [unwired: 2 in, 2 out]
                      }
                      frame #1 {
                        n284 = Bundle("Minimum"=-5.0, "Minimum"=37.3, "Minimum"=10.0, "Minimum"=1.0, "Minimum"=-20.0) -> (w376:T13)  [unwired: 1 in]
                        n285 = Bundle("Minimum"=-22.6, "Minimum"=22.6, "Minimum"=10.0, "Minimum"=1.0, "Minimum"=-20.0) -> (w383:T13)  [unwired: 1 in]
                        n286 = property on="XY Graph" class="XYGraph (strict)"("YScale.Range"=w376) -> ()  [unwired: 2 in, 2 out]
                        n287 = property on="XY Graph" class="XYGraph (strict)"("XScale.Range"=w383) -> ()  [unwired: 2 in, 2 out]
                      }
                      frame #2 {
                        n288 = global read "G_DATA.vi" "path"() -> (w387:path)
                        n289 = Build Path(base path=w387, name or relative path="wpt") -> (appended path=w385:path)
                        n290 = call "Read From Measurement File2"("Filename"=w385, "Reset"=TRUE) -> ("error out"=w389:errorcluster, "Filename Out"=w384:path, "Signals"=w391:dynamicdata)  [unwired: 4 in, 3 out]
                        n291 = Unbundle By Name(w389) -> ("status"=w388:bool)
                        n292 = case shown="False" w388 {
                          tunnel: w391 -> [w393 _]
                          tunnel: w384 -> [w392 _]
                          frame False {
                            n293 = call "Convert from Dynamic Data2"("Dynamic Data Type"=w393) -> ("Array"=w395:dbl[][])  [unwired: 3 in]
                            n294 = Empty Array?(array=w395) -> (empty?=w394:bool)
                            n295 = case shown="False" w394 {
                              tunnel: w395 -> [w397 _]
                              tunnel: w392 -> [w396 _]
                              frame False {
                                n296 = call "path_ini_new.vi"("Filename Out"=w396, "WPT"=w397) -> ()  [unwired: 10 in]
                              }
                              frame True {
                                w398 = dbl[][] [] ("path_updated")
                                n297 = global write "G_PATH.vi" "path"(w398) -> ()
                                n298 = global write "G_PATH.vi" "path_very_origin"(w398) -> ()
                                n299 = global write "G_PATH.vi" "path_origin"(w398) -> ()
                              }
                            }
                          }
                          frame True {
                            w399 = dbl[][] [] ("path_updated")
                            n300 = global write "G_PATH.vi" "path"(w399) -> ()
                            n301 = global write "G_PATH.vi" "path_very_origin"(w399) -> ()
                            n302 = global write "G_PATH.vi" "path_origin"(w399) -> ()
                          }
                        }
                      }
                      frame #3 {
                        w400 = T14 [] ("Missions_origin")
                        n303 = global read "G_VEH.vi" "Location"() -> (w401:i32)
                        n304 = local write "Load Path"(FALSE ("Load WPT")) -> ()
                        n305 = global write "G_PATH.vi" "Missions_origin"(w400) -> ()
                        n306 = global write "G_PATH.vi" "Missions"(w400) -> ()
                        n307 = call "mapconf.vi"("Location"=w401) -> ("y"=w403:cluster{dbl, dbl, "y":dbl, "y":dbl, dbl}, "x"=w404:cluster{dbl, dbl, "y":dbl, "y":dbl, dbl}, "new picture"=w405:picture)  [unwired: 8 in]
                        n308 = property on="XY Graph 2" class="XYGraph (strict)"("PlotImages.Back"=w405) -> ()  [unwired: 2 in, 2 out]
                        n309 = property on="XY Graph 2" class="XYGraph (strict)"("XScale.Range"=w404, "YScale.Range"=w403) -> ()  [unwired: 2 in, 2 out]
                      }
                    }
                  }
                }
              }
              frame True {
                n310 = flat-sequence {
                  tunnel: [w410] -> w406
                  tunnel: w406 -> [w499]
                  frame #0 {
                    w407 = 0.0
                    n311 = global write "G_VEH.vi" "handle"(w407) -> ()
                    n312 = global write "G_VEH.vi" "VS_des"(w407) -> ()
                  }
                  frame #1 {
                    n313 = local read "Make WPT"() -> (w409:bool)
                    n314 = global read "G_VEH.vi" "Location"() -> (w408:i32)
                    n315 = Initialize Array(0.0 ("element"), 7 ("dimension size"), 1 ("dimension size")) -> (w411:dbl[][])
                    n316 = while {
                      shift-right: [w416] -> w410
                      shift-left: w411 -> [w418]
                      shift-right: [FALSE] -> _
                      shift-left: w409 -> [w419]
                      tunnel: w408 -> [w415]
                      stop <- w421 stop-if-true
                      n317 = local read "Make WPT"() -> (w422:bool)
                      n318 = flat-sequence {
                        tunnel: [w431] -> w417
                        tunnel: w415 -> [w424]
                        frame #0 {
                          n319 = global read "G_NAV.vi" "GPS_status"() -> (w423:T15)
                          n320 = disable-structure shown="Enabled" {
                            disable-tunnel: [w442 w446] -> w434
                            disable-tunnel: [w441 w445] -> w433
                            disable-tunnel: [w435 w444] -> w432
                            disable-tunnel: w423 -> [w440 w454]
                            disable-tunnel: [w439 w453] -> w430
                            disable-tunnel: [w438 w452] -> w429
                            disable-tunnel: [w435 w451] -> w428
                            disable-tunnel: w424 -> [_ w450]
                            frame Enabled {
                              n321 = Unbundle By Name(w440) -> ("lat"=w439:dbl, "lon"=w438:dbl, "hgt"=w435:dbl)
                              n322 = global read "G_NAV.vi" "M6006"() -> (w443:T12)
                              n323 = Unbundle By Name(w443) -> ("lcc[0]"=w437:dbl, "lcc[1]"=w436:dbl)
                              n324 = To Double Precision Float(number=w437) -> (double precision float=w442:dbl)
                              n325 = To Double Precision Float(number=w436) -> (double precision float=w441:dbl)
                            }
                            frame Disabled {
                              n326 = Unbundle By Name(w454) -> ("lat"=w453:dbl, "lon"=w452:dbl, "hgt"=w451:dbl)
                              n327 = call "getecefdcmref.vi"("map"=w450) -> ("XYZ"=w449:dbl[])  [unwired: 10 in, 4 out]
                              n328 = call "llh2lcc.vi"("ecef ref"=w449, "hgt"=w451, "lon"=w452, "lat"=w453) -> ("lcc"=w448:dbl[])  [unwired: 7 in]
                              n329 = Index Array(array=w448, index #1=0 ("index")) -> (element #1=w446:dbl, element #2=w445:dbl, element #3=w444:dbl)  [unwired: 2 in]
                            }
                          }
                          n330 = To Double Precision Float(number=w424) -> (double precision float=w425:dbl)
                          n331 = global read "G_VEH.vi" "candata"() -> (w427:T8)
                          n332 = Unbundle By Name(w427) -> ("VS_can"=w426:dbl)
                          n333 = Build Array(w430, w429, w428, w434, w433, w432, w426, w425) -> (w431:dbl[])
                        }
                      }
                      n334 = Not(x=w422) -> (.not. x?=w421:bool)
                      n335 = case shown="False" w419 {
                        tunnel: w418 -> [w469 w486]
                        tunnel: w417 -> [w468 w484]
                        tunnel: [w467 w483] -> w416
                        frame False {
                          n336 = Array Size(array=w469) -> (size(s)=w477:i32[])
                          n337 = Index Array(array=w468, index #1=3 ("index"), index #2=4 ("index")) -> (element #1=w463:dbl, element #2=w461:dbl)
                          n338 = Index Array(array=w477, index=1) -> (element=w466:i32)
                          n339 = Decrement(x=w466) -> (x-1=w465:i32)
                          n340 = Index Array(array=w469, index (col)=w465) -> (element=w473:dbl[])  [unwired: 1 in]
                          n341 = Index Array(array=w473, index #1=3 ("index"), index #2=4 ("index")) -> (element #1=w464:dbl, element #2=w462:dbl)
                          n342 = Subtract(x=w464, y=w463) -> (x-y=w460:dbl)
                          n343 = Subtract(x=w462, y=w461) -> (x-y=w459:dbl)
                          n344 = Square(x=w460) -> (x^2=w458:dbl)
                          n345 = Square(x=w459) -> (x^2=w457:dbl)
                          n346 = Add(x=w458, y=w457) -> (x+y=w456:dbl)
                          n347 = Greater Or Equal?(x=w456, y=0.25) -> (x >= y?=w470:bool)
                          n348 = case shown="True" w470 {
                            tunnel: w469 -> [w478 w482]
                            tunnel: w466 -> [_ w479]
                            tunnel: w468 -> [_ w481]
                            tunnel: [w478 w480] -> w467
                            frame False {
                            }
                            frame True {
                              n349 = Insert Into Array(array=w482, index (col)=w479, new element=w481) -> (w480:dbl[][])  [unwired: 1 in]
                            }
                          }
                        }
                        frame True {
                          n350 = Replace Array Subset(array=w486, new element=w484, index (col)=0 ("disabled index (col)")) -> (w483:dbl[][])  [unwired: 1 in]
                        }
                      }
                    }
                  }
                  frame #2 {
                    n351 = call "Convert to Dynamic Data"("2D Array"=w499) -> ("Dynamic Data Type"=w500:dynamicdata)  [unwired: 3 in]
                    n352 = global read "G_VEH.vi" "Location"() -> (w496:i32)
                    n353 = case shown="9" w496 {
                      tunnel: ["" ("String") "Hyundai" ("String") "KAIST" ("String") "AJOU" ("String") "MUNJI" ("String") "Airforce" ("String") "CAR" ("String") "KATRI" ("String") _ "coex" ("String")] -> w495
                      frame 0, Default {
                      }
                      frame 1 {
                      }
                      frame 2 {
                      }
                      frame 3 {
                      }
                      frame 4 {
                      }
                      frame 5 {
                      }
                      frame 6 {
                      }
                      frame 7 {
                      }
                      frame 8 {
                      }
                      frame 9 {
                      }
                    }
                    n354 = Get Date/Time In Seconds() -> (seconds since 1Jan1904=w497:timestamp)
                    n355 = Format Date/Time String(time format string (%c)="%2y%2m%2d%2H%2M", seconds (now)=w497) -> (date/time string=w493:string)  [unwired: 1 in]
                    n356 = global read "G_DATA.vi" "path"() -> (w491:path)
                    n357 = Build Path(base path=w491, name or relative path="wpt") -> (appended path=w489:path)
                    n358 = Concatenate Strings(w493, "_" ("string"), w495, ".lvm" ("string")) -> (w488:string)
                    n359 = Build Path(base path=w489, name or relative path=w488) -> (appended path=w487:path)
                    n360 = call "save wpt"("Signals"=w500, "Reset"=TRUE, "Filename"=w487) -> ()  [unwired: 14 in, 3 out]
                  }
                }
              }
            }
          }
        }
      }
    }
  }
  n361 = flat-sequence {
    frame #0 {
      # "Sensor paser"
    }
    frame #1 {
      n362 = local write "Log"(FALSE ("obs")) -> ()
    }
    frame #2 {
      n363 = while {
        stop <- FALSE ("Loop 4") stop-if-true
        n364 = flat-sequence {
          frame #0 {
            n365 = Wait Until Next ms Multiple(millisecond multiple=u32 10 ("milliseconds to wait")) -> (millisecond timer value=w513:u32)
            n366 = feedback #7() -> (w515:u32)  [unwired: 1 in]
            n367 = feedback-in #7(w513) -> ()
            n368 = Subtract(x=w513, y=w515) -> (x-y=→"sensor":u32)
          }
          frame #1 {
            n369 = disable-structure shown="Enabled" {
              frame Disabled {
                w548 = 0.0 ("roll")
                n370 = call "velodynepaser.vi"("roll"=w548, "pitch"=w548, "heading"=w548, "dX"=w548, "dY"=w548, "dZ"=w548) -> ()  [unwired: 12 in, 2 out]
              }
              frame Enabled {
              }
            }
            n371 = global read "G_LCM.vi" "Mobileye name"() -> (w517:string)
            n372 = case shown="\"Mobileye560\"" w517 {
              frame Default {
                n373 = call "mobileyelanepaser4.vi"("count hold"=u64 15, "thresh  c"=0.5, "thresh  b"=0.06 ("thresh 2"), "thresh r"=0.009 ("y")) -> ()  [unwired: 4 in, 4 out]
                n374 = call "mobileyepaser.vi"() -> ()  [unwired: 11 in, 1 out]
              }
              frame "Mobileye560" {
                n375 = global read "G_LCM.vi" "Mobileye_RAW_SNAP"() -> (w522:T17)
                n376 = Unbundle By Name(w522) -> ("size"=w523:i32, "data"=w526:u8[])
                n377 = Divide(x=w523, y=16) -> (x/y=w525:dbl)
                n378 = for {
                  N: w525 -> [_]
                  tunnel: w526 -> [w546]
                  i -> [w545]
                  w538 = 4 ("length")
                  w536 = 8 ("index")
                  w544 = 16 ("y")
                  n379 = Multiply(x=w545, y=w544) -> (x*y=w543:i32)
                  n380 = Array Subset(array=w546, index=w543, length=w544) -> (w528:u8[])
                  n381 = Delete From Array(array=w528, length=w536, index=w536) -> (deleted portion=w529:u8[], array with subset deleted=w537:u8[])
                  n382 = Delete From Array(array=w537, length=w538, index=w538) -> (deleted portion=w542:u8[], array with subset deleted=w539:u8[])
                  n383 = Type Cast(type=u32 0, x=w539) -> (*(type *) &x=w530:u32)
                  n384 = Type Cast(type=u32 0, x=w542) -> (*(type *) &x=w531:u32)
                  n385 = Multiply(x=w531, y=1e-07) -> (x*y=w534:dbl)
                  n386 = To Time Stamp(1:w534) -> (0:w533:timestamp)
                  n387 = global read "G_LCM.vi" "Mobileye name"() -> (w547:string)
                  n388 = Bundle By Name(cluster=T16 {"identifier"=0, "timestamp"=timestamp(0 s since 1904-01-01), "payload"=[]} ("can cluster"), "identifier"=w530, "payload"=w529, "timestamp"=w533) -> (w527:T16)
                  n389 = call "mobileye_decoder_PC.vi"("can cluster"=w527, "name"=w547) -> ()  [unwired: 10 in]
                }
              }
            }
          }
          frame #2 {
            w551 = TRUE ("Sensor [F12]")
            n390 = global read "G_SEN.vi" "M_lane_update"() -> (→"update":bool)
            n391 = call "Ibeopaser.vi"("theta"=-2.5, "Hide Transparent"=w551, "Sensor [F12]"=w551) -> ("x_sensor"=w555:T6, "etc"=w553:dbl[][], "lane"=w554:dbl[][], "obs"=w556:dbl[][], "update"=w552:bool)  [unwired: 4 in]
            n392 = case shown="True" w552 {
              tunnel: w556 -> [_ w561]
              tunnel: w555 -> [_ w562]
              tunnel: w554 -> [_ w558]
              tunnel: w553 -> [_ w559]
              frame False {
              }
              frame True {
                n393 = disable-structure shown="Enabled" {
                  disable-tunnel: w561 -> [w567 w569]
                  disable-tunnel: [w566 w569] -> w560
                  disable-tunnel: w559 -> [w565 _]
                  disable-tunnel: w558 -> [w564 w568]
                  disable-tunnel: [w563 w568] -> w557
                  frame Disabled {
                    n394 = call "test3.vi"("sensor_all"=w565, "sensor_lane"=w564, "sensor_obs"=w567) -> ("lane"=w563:dbl[][], "obs"=w566:dbl[][])  [unwired: 6 in, 1 out]
                  }
                  frame Enabled {
                  }
                }
                n395 = global write "G_VEH.vi" "xsensor"(w562) -> ()
                n396 = global write "G_SEN.vi" "sensor_obs"(w560) -> ()
                n397 = global write "G_SEN.vi" "sensor_lane"(w557) -> ()
              }
            }
          }
          frame #3 {
            n398 = case shown="True" "Log" {
              frame False {
                n399 = global write "G_SEN.vi" "sensor_obs_log"(dbl[][] [] ("sensor_obs_log")) -> ()
              }
              frame True {
                n400 = global read "G_VEH.vi" "candata"() -> (w573:T8)
                n401 = Unbundle By Name(w573) -> ("VS_can"=w574:dbl)
                n402 = Not Equal To 0?(x=w574) -> (x != 0?=w572:bool)
                n403 = case shown="True" w572 {
                  frame False {
                  }
                  frame True {
                    n404 = global read "G_SEN.vi" "sensor_obs_log"() -> (w576:dbl[][])
                    n405 = global read "G_SEN.vi" "sensor_obs"() -> (w577:dbl[][])
                    n406 = call "sensor_log2.vi"("xmax"=8.0, "range^2"=16.0, "xmin"=-5.0, "FF"=0.93 ("t"), "ymin"=0.0, "ymax"=20.0, "sensor_log"=w576, "sensor_obs"=w577) -> ("sensor_log 2"=w575:dbl[][])  [unwired: 2 in, 1 out]
                    n407 = global write "G_SEN.vi" "sensor_obs_log"(w575) -> ()
                  }
                }
              }
            }
          }
          frame #4 {
            n408 = disable-structure shown="Enabled" {
              frame Disabled {
                n409 = global read "G_VEH.vi" "candata"() -> (w590:T8)
                n410 = global read "G_VEH.vi" "sys time"() -> (w585:i64)
                n411 = Unbundle By Name(w590) -> ("VS_can"=w591:dbl)
                n412 = feedback-in #8(w585) -> ()
                n413 = feedback #8(i64 0 ("sys time")) -> (w589:i64)
                n414 = Not Equal To 0?(x=w591) -> (x != 0?=w587:bool)
                n415 = Greater?(x=w585, y=w589) -> (0:w588:bool)
                n416 = And(x=w587, y=w588) -> (x .and. y?=w586:bool)
                n417 = case shown="True" w586 {
                  frame False {
                  }
                  frame True {
                    n418 = flat-sequence {
                      tunnel: [w593] -> w592
                      tunnel: w592 -> [w611]
                      frame #0 {
                        n419 = disable-structure shown="Enabled" {
                          disable-tunnel: [50.0 ("ymax") 10000.0 ("ymax")] -> w598
                          disable-tunnel: [-3.5 ("ymin") -10000.0 ("ymin")] -> w597
                          disable-tunnel: [-6.0 ("xmin") -10000.0 ("xmin")] -> w596
                          disable-tunnel: [10.0 ("xmin") 10000.0 ("xmax")] -> w595
                          frame Enabled {
                          }
                          frame Disabled {
                          }
                        }
                        n420 = global read "G_SEN.vi" "sensor_lane_log"() -> (w602:dbl[][])
                        n421 = global read "G_SEN.vi" "sensor_lane"() -> (w601:dbl[][])
                        n422 = call "sensor_log2.vi"("xmax"=w595, "range^2"=0.0, "xmin"=w596, "FF"=1.0, "ymin"=w597, "ymax"=w598, "sensor_log"=w602, "sensor_obs"=w601) -> ("sensor_log_body"=w593:dbl[][], "sensor_log 2"=w594:dbl[][])  [unwired: 2 in]
                        n423 = global write "G_SEN.vi" "sensor_lane_log"(w594) -> ()
                      }
                      frame #1 {
                        n424 = disable-structure shown="Enabled" {
                          disable-tunnel: w611 -> [w612 _]
                          frame Disabled {
                            n425 = call "lane_test1.vi"("lane_body"=w612) -> ()  [unwired: 11 in]
                          }
                          frame Enabled {
                          }
                        }
                      }
                    }
                  }
                }
              }
              frame Enabled {
              }
            }
          }
        }
      }
    }
  }
